vi "test.1.vi"(11 "Inputs":bool) -> (3 "Results":bool)   [LabVIEW 2020]
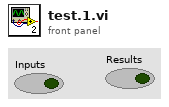
[diagram p1: front panel]
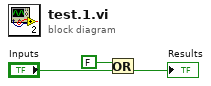
[diagram p0: block diagram]
diagram:
  n1 = Or(x=FALSE, y="Inputs") -> (x .or. y?=→"Results":bool)
